vi "Plane.vi"() -> ()   [LabVIEW 2012]
panel:
  out "Z Plane":cluster{"X":dbl, "Y":dbl}[](graph)
  out "S Plane":cluster{"X":dbl, "Y":dbl}[](graph)
  out "Nychols":cluster{"X":dbl, "Y":dbl}[](graph)
  out "Nyquist":cluster{"X":dbl, "Y":dbl}[](graph)
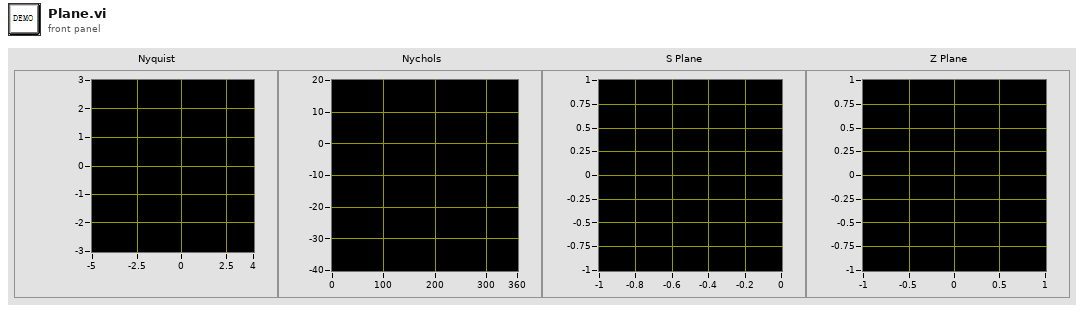
[diagram p1: front panel]
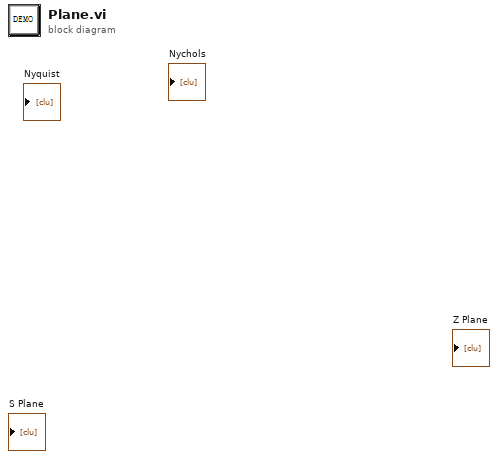
[diagram p0: block diagram]
diagram:
